vi "Hardware PID Controller.vi"(6 "Simulate":bool, 7 "Simulated Actual Pressure":dbl, 8 "error in (no error)":errorcluster, 10 "DAQ Ref Cluster in":T3, 11 "State Machine Data":T1={"Control State"="", "Status Message"="", "Speed"=0.0, "Pressure"=0.0, "Target Pressure"=0.0, "Apply Brake Ref"=refnum, "Release Brake Ref"=refnum, "Extend Ref"=refnum, "Retract Ref"=refnum, "Pressure Ref"=refnum, "Data Display Ref"=refnum, "Exit Button Ref"=refnum, "Bool"=TRUE, "Status"={"Extend"=FALSE, "Brake"=FALSE, "Retract"=FALSE}}) -> (0 "error out":errorcluster, 2 "DAQ Ref Cluster out":T3, 3 "Data Cluster out":T4)   [LabVIEW 2021]
uses:
  Controls/UI Data.ctl
  Controls/Status Lights.ctl
  Controls/DAQ Refnums.ctl
  Controls/State Machine Data.ctl
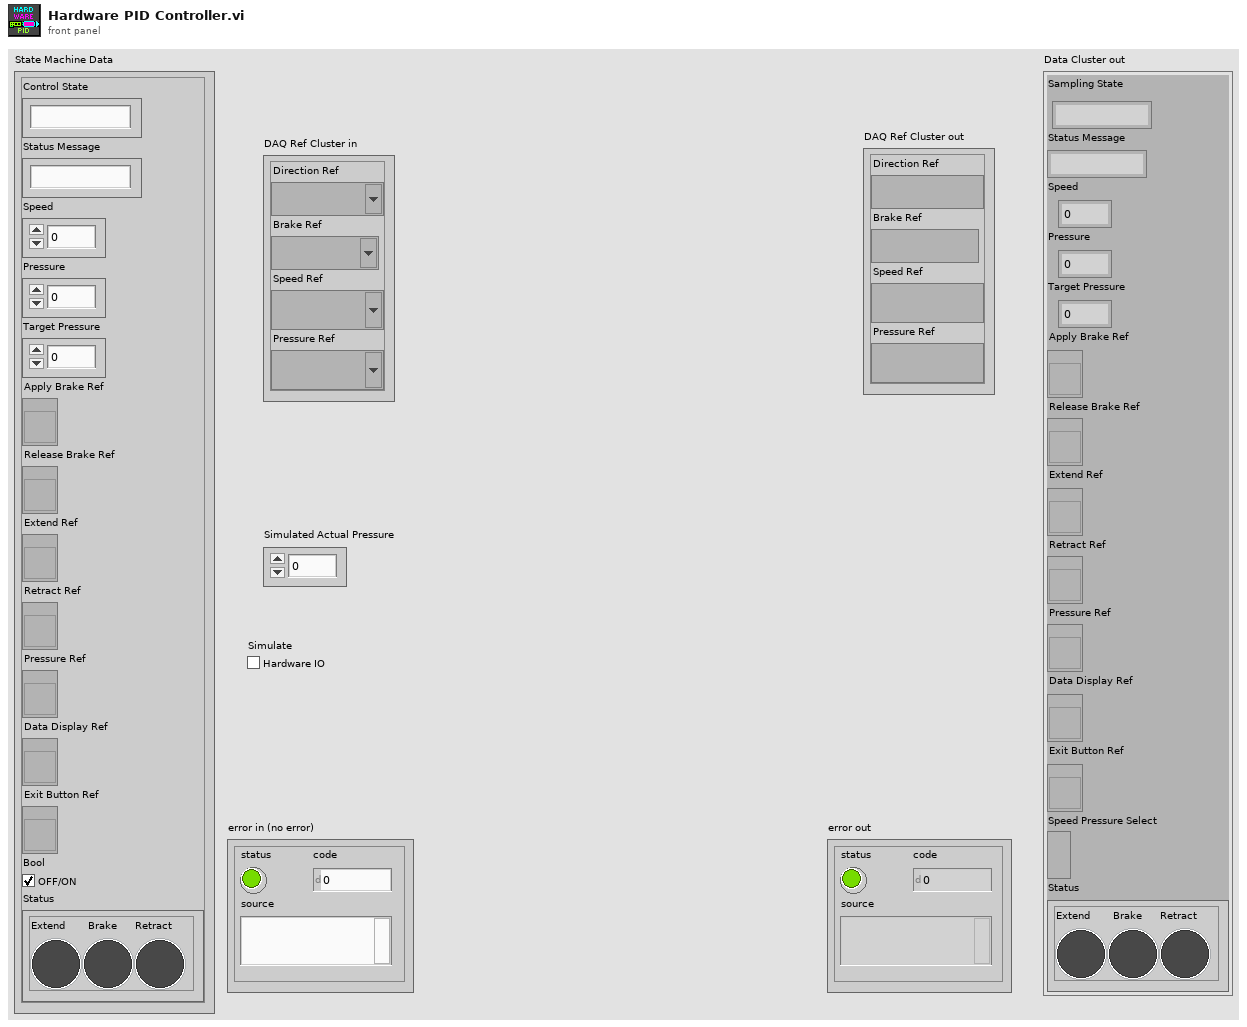
[diagram p1: front panel]
types:
  T1 = typedef "State Machine Data.ctl" = cluster{"Control State":string, "Status Message":string, "Speed":dbl, "Pressure":dbl, "Target Pressure":dbl, "Apply Brake Ref":refnum<vi>, "Release Brake Ref":refnum<vi>, "Extend Ref":refnum<vi>, "Retract Ref":refnum<vi>, "Pressure Ref":refnum<vi>, "Data Display Ref":refnum<vi>, "Exit Button Ref":refnum<vi>, "Bool":bool, "Status":T2}
  T2 = typedef "Status Lights.ctl" = cluster{"Extend":bool, "Brake":bool, "Retract":bool}
  T3 = typedef "DAQ Refnums.ctl" = cluster{"Direction Ref":refnum<k21>, "Brake Ref":refnum<k21>, "Speed Ref":refnum<k21>, "Pressure Ref":refnum<k21>}
  T4 = typedef "UI Data.ctl" = cluster{"Sampling State":string, "Status Message":string, "Speed":dbl, "Pressure":dbl, "Target Pressure":dbl, "Apply Brake Ref":refnum<vi>, "Release Brake Ref":refnum<vi>, "Extend Ref":refnum<vi>, "Retract Ref":refnum<vi>, "Pressure Ref":refnum<vi>, "Data Display Ref":refnum<vi>, "Exit Button Ref":refnum<vi>, "Speed Pressure Select":bool, "Status":T2}
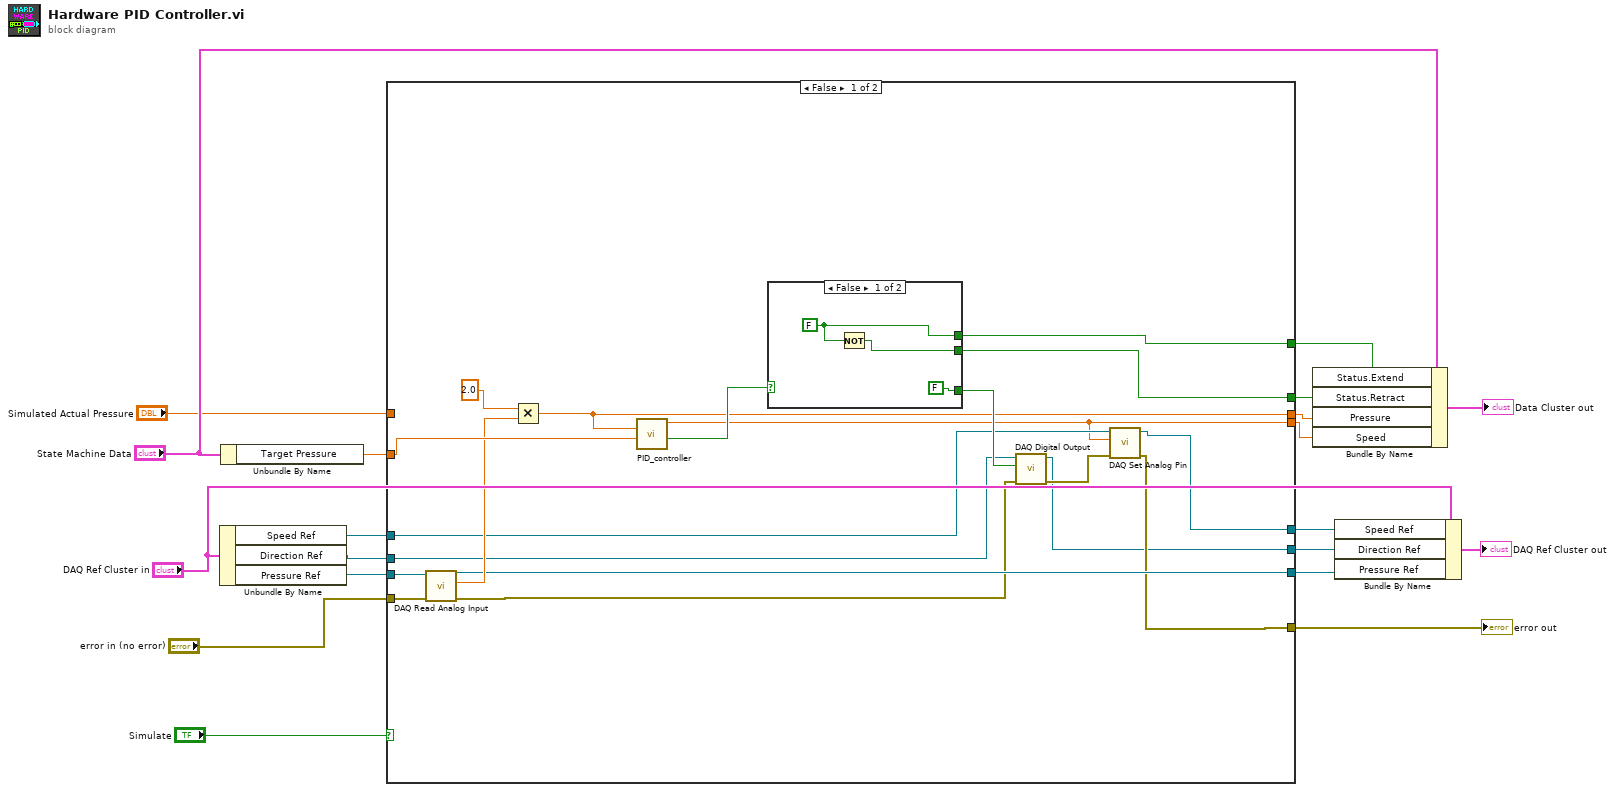
[diagram p0: block diagram]
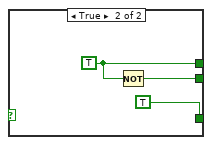
[diagram p2: hidden frame]
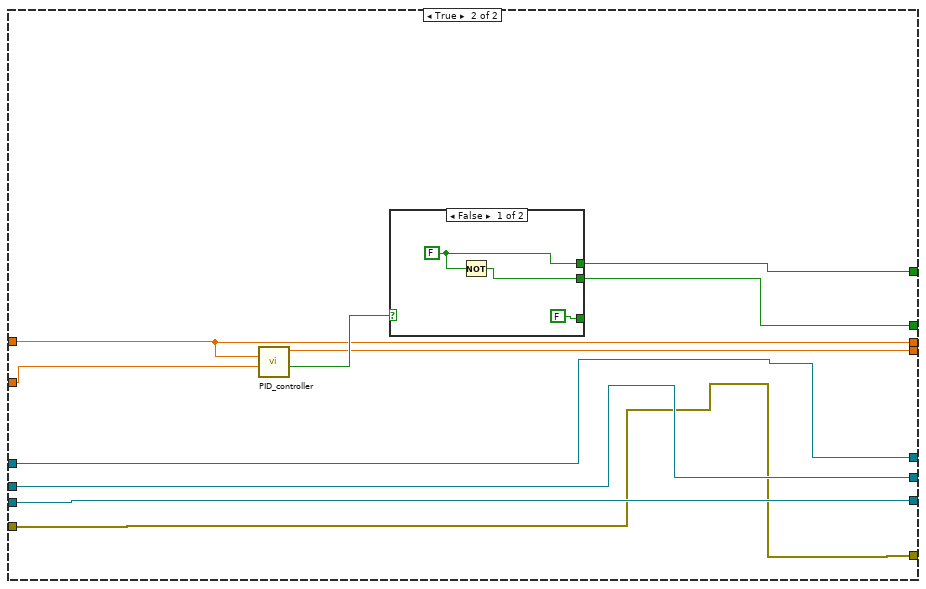
[diagram p3: hidden frame]
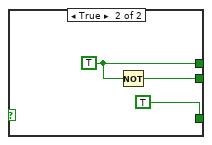
[diagram p4: hidden frame]
diagram:
  n1 = Unbundle By Name("DAQ Ref Cluster in") -> ("Speed Ref"=w9:refnum<k21>, "Direction Ref"=w11:refnum<k21>, "Pressure Ref"=w13:refnum<k21>)
  n2 = Unbundle By Name("State Machine Data") -> ("Target Pressure"=w19:dbl)
  n3 = case shown="False" "Simulate" {
    tunnel: w19 -> [w38 w54]
    tunnel: "error in (no error)" -> [w37 w45]
    tunnel: [w35 w49] -> w17
    tunnel: w13 -> [w34 w49]
    tunnel: [w29 w45] -> w12
    tunnel: w11 -> [w28 w47]
    tunnel: [w27 w47] -> w10
    tunnel: w9 -> [w26 w46]
    tunnel: [w25 w46] -> w8
    tunnel: [w23 w52] -> w7
    tunnel: [w22 w48] -> w6
    tunnel: [w21 w51] -> w4
    tunnel: [w20 w50] -> w3
    tunnel: "Simulated Actual Pressure" -> [_ w48]
    frame False {
      n4 = call "DAQ Read Analog Input.vi"("error in"=w37, "task/channels in"=w34) -> ("error out"=w31:errorcluster, "Voltage"=w36:dbl, "task out"=w35:refnum<k21>)  [unwired: 7 in]
      n5 = Multiply(x=2.0, y=w36) -> (x*y=w22:dbl)
      n6 = call "PID_controller.vi"("Setpoint"=w38, "Process Variable"=w22) -> ("Direction"=w33:bool, "output"=w23:dbl)  [unwired: 6 in, 2 out]
      n7 = case shown="False" w33 {
        tunnel: [FALSE ("data") TRUE ("data")] -> w32
        tunnel: [w39 w43] -> w21
        tunnel: [w40 w42] -> w20
        frame False {
          w39 = FALSE ("Status.Extend")
          n8 = Not(x=w39) -> (.not. x?=w40:bool)
        }
        frame True {
          w43 = TRUE ("Status.Extend")
          n9 = Not(x=w43) -> (.not. x?=w42:bool)
        }
      }
      n10 = call "DAQ Digital Output.vi"("error in"=w31, "data"=w32, "task/channels in"=w28) -> ("error out"=w30:errorcluster, "task out"=w27:refnum<k21>)  [unwired: 6 in, 1 out]
      n11 = call "DAQ Set Analog Pin.vi"("error in"=w30, "Voltage"=w23, "task/channels in"=w26) -> ("error out"=w29:errorcluster, "task out"=w25:refnum<k21>)  [unwired: 6 in, 1 out]
    }
    frame True {
      n12 = call "PID_controller.vi"("Setpoint"=w54, "Process Variable"=w48) -> ("Direction"=w53:bool, "output"=w52:dbl)  [unwired: 6 in, 2 out]
      n13 = case shown="False" w53 {
        tunnel: [FALSE ("data") TRUE ("data")] -> _
        tunnel: [w55 w59] -> w51
        tunnel: [w56 w58] -> w50
        frame False {
          w55 = FALSE ("Status.Extend")
          n14 = Not(x=w55) -> (.not. x?=w56:bool)
        }
        frame True {
          w59 = TRUE ("Status.Extend")
          n15 = Not(x=w59) -> (.not. x?=w58:bool)
        }
      }
    }
  }
  "error out" <- w12
  n16 = Bundle By Name(cluster="State Machine Data", "Status.Extend"=w4, "Status.Retract"=w3, "Pressure"=w6, "Speed"=w7) -> (→"Data Cluster out":T1)
  n17 = Bundle By Name(cluster="DAQ Ref Cluster in", "Speed Ref"=w8, "Direction Ref"=w10, "Pressure Ref"=w17) -> (→"DAQ Ref Cluster out":T3)
